vi "Query & Delete RTSeq Test Data.vi"(8 "Error In":errorcluster, 11 "RT Seq Ref In":refnum<k24>) -> (0 "Error Out":errorcluster, 1 "Parameters":refnum<k24>[](array[refnum]), 3 "RT Seq Ref Out":refnum<k24>, 5 "1 CSVs Tests":T1)   [LabVIEW 2011]
uses:
  NationalInstruments.VeriStand.RealTimeSequenceDefinitionApi
  Controls/CSVs Tests Data.ctl
  Controls/Test Column Data.ctl
  NationalInstruments.VeriStand.DataTypes
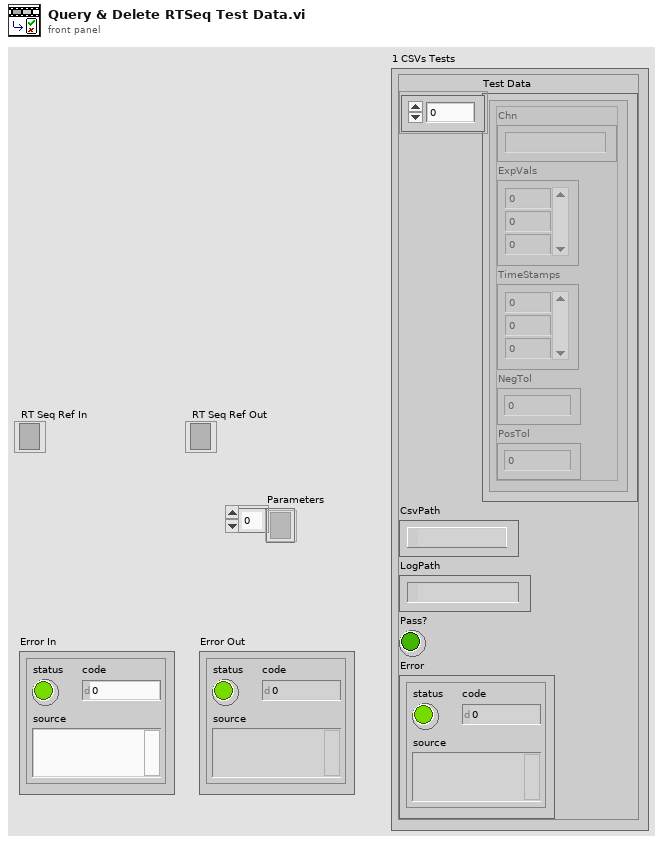
[diagram p1: front panel]
types:
  T1 = typedef "CSVs Tests Data.ctl" = cluster{"Test Data":T2[], "CsvPath":path, "LogPath":path, "Pass?":bool, "Error":errorcluster}
  T2 = typedef "Test Column Data.ctl" = cluster{"Chn":string, "ExpVals":dbl[], "TimeStamps":i64[], "NegTol":dbl, "PosTol":dbl}
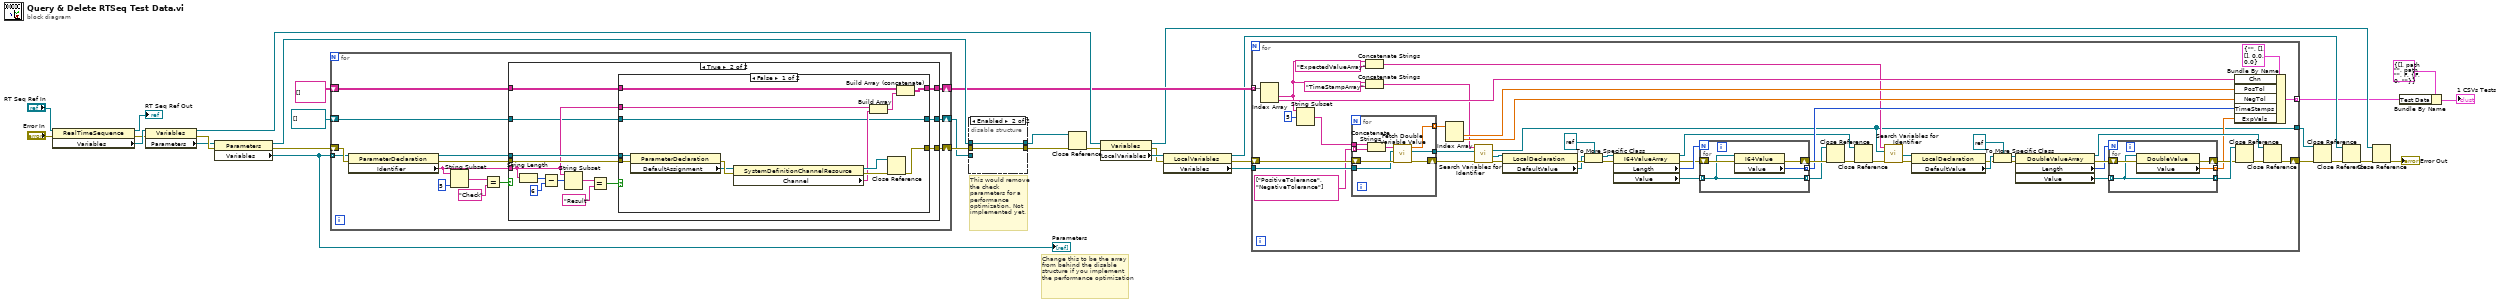
[diagram p0: block diagram]
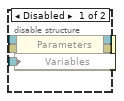
[diagram p2: hidden frame]
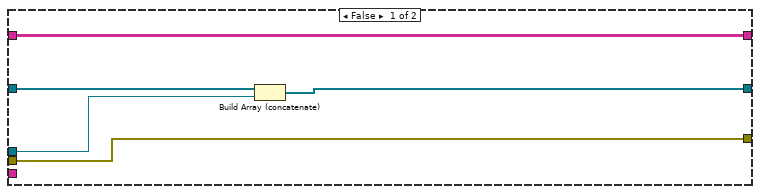
[diagram p3: hidden frame]
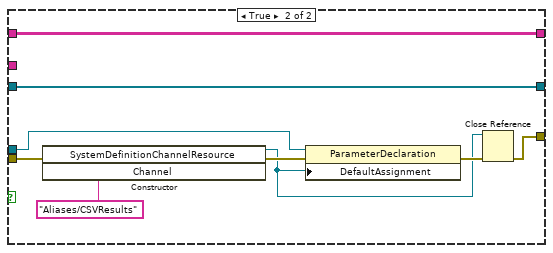
[diagram p4: hidden frame]
diagram:
  # "Change this to be the array from behind the disable structure if you implement the performance optimization"
  # "This would remove the check parameters for a performance optimization. Not implemented yet."
  n1 = property class="RealTimeSequence"(reference="RT Seq Ref In", error in="Error In") -> (reference out=→"RT Seq Ref Out":refnum<k24>, error out=w32:errorcluster, "Variables"=w33:refnum<k24>)
  n2 = property class="Variables"(reference=w33, error in=w32) -> (reference out=w17:refnum<k24>, error out=w28:errorcluster, "Parameters"=w25:refnum<k24>)
  n3 = property class="Parameters"(reference=w25, error in=w28) -> (reference out=w21:refnum<k24>, error out=w27:errorcluster, "Variables"=w20:refnum<k24>[])
  "Parameters" <- w20
  n4 = for {
    tunnel: w20 -> [w46] mode=indexing
    shift-right: [w34] -> w23
    shift-left: w27 -> [w47]
    shift-right: [w37] -> w16
    shift-left: string[][] [] -> [w38]
    shift-right: [w35] -> w22
    shift-left: refnum<k24>[] [] -> [w36]
    n5 = property class="ParameterDeclaration"(reference=w46, error in=w47) -> (reference out=w40:refnum<k24>, error out=w42:errorcluster, "Identifier"=w39:string)
    n6 = String Subset(string=w39, length (rest)=5 ("length (rest)")) -> (substring=w44:string)  [unwired: 1 in]
    n7 = Equal?(x=w44, y="Check") -> (x = y?=w41:bool)
    n8 = case shown="True" w41 {
      tunnel: w42 -> [w51 w60]
      tunnel: w40 -> [w49 w59]
      tunnel: w39 -> [_ w56]
      tunnel: w38 -> [w52 w58]
      tunnel: [w52 w57] -> w37
      tunnel: w36 -> [w50 w55]
      tunnel: [w48 w54] -> w35
      tunnel: [w51 w53] -> w34
      frame False {
        n9 = Build Array (concatenate)(w50, w49) -> (w48:refnum<k24>[])
      }
      frame True {
        n10 = String Length(string=w56) -> (length=w66:i32)
        n11 = Subtract(x=w66, y=6) -> (x-y=w64:i32)
        n12 = String Subset(string=w56, offset (0)=w64) -> (substring=w63:string)  [unwired: 1 in]
        n13 = Equal?(x=w63, y="Result") -> (x = y?=w61:bool)
        n14 = case shown="False" w61 {
          tunnel: w60 -> [w79 w86]
          tunnel: w59 -> [w78 w84]
          tunnel: w58 -> [w75 w88]
          tunnel: [w74 w88] -> w57
          tunnel: [w71 w80] -> w53
          tunnel: w56 -> [w69 _]
          tunnel: w55 -> [w67 w87]
          tunnel: [w67 w87] -> w54
          frame False {
            n15 = property class="ParameterDeclaration"(reference=w78, error in=w79) -> (error out=w77:errorcluster, "DefaultAssignment"=w76:refnum<k24>)  [unwired: 1 out]
            n16 = property class="SystemDefinitionChannelResource"(reference=w76, error in=w77) -> (reference out=w72:refnum<k24>, error out=w73:errorcluster, "Channel"=w68:string)
            n17 = Build Array(w69, w68) -> (w70:string[])
            n18 = Close Reference(reference=w72, error in (no error)=w73) -> (error out=w71:errorcluster)
            n19 = Build Array (concatenate)(w75, w70) -> (w74:string[][])
          }
          frame True {
            n20 = constructor class="SystemDefinitionChannelResource"(error in=w86, "Channel"="Aliases/CSVResults" ("y")) -> (reference out=w81:refnum<k24>, error out=w85:errorcluster)  [unwired: 2 in, 2 out]
            n21 = property class="ParameterDeclaration"(reference=w84, error in=w85, "DefaultAssignment"=w81) -> (error out=w82:errorcluster)  [unwired: 1 out]
            n22 = Close Reference(reference=w81, error in (no error)=w82) -> (error out=w80:errorcluster)
          }
        }
      }
    }
  }
  n23 = disable-structure shown="Enabled" {
    disable-tunnel: w23 -> [w93 w95]
    disable-tunnel: w22 -> [w92 _]
    disable-tunnel: w21 -> [w91 w94]
    disable-tunnel: [w90 w95] -> w4
    disable-tunnel: [w89 w94] -> w19
    frame Disabled {
      n24 = property class="Parameters"(reference=w91, error in=w93, "Variables"=w92) -> (reference out=w89:refnum<k24>, error out=w90:errorcluster)
    }
    frame Enabled {
    }
  }
  n25 = Close Reference(reference=w19, error in (no error)=w4) -> (error out=w18:errorcluster)
  n26 = property class="Variables"(reference=w17, error in=w18) -> (reference out=w6:refnum<k24>, error out=w14:errorcluster, "LocalVariables"=w15:refnum<k24>)
  n27 = property class="LocalVariables"(reference=w15, error in=w14) -> (reference out=w7:refnum<k24>, error out=w12:errorcluster, "Variables"=w13:refnum<k24>[])
  n28 = for {
    tunnel: w16 -> [w146] mode=indexing
    tunnel: w13 -> [w144]
    shift-right: [w97] -> w11
    shift-left: w12 -> [w147]
    tunnel: [w130] -> w2 mode=indexing
    tunnel: [w96] -> w10
    n29 = Index Array(array=w146) -> (element #1=w131:string, element #2=w142:string)  [unwired: 2 in]
    n30 = String Subset(string=w131, offset (0)=5) -> (substring=w141:string)  [unwired: 1 in]
    n31 = for {
      tunnel: w144 -> [w161]
      tunnel: w141 -> [w160]
      shift-right: [w158] -> w136
      shift-left: w147 -> [w163]
      tunnel: string[] ["PositiveTolerance", "NegativeTolerance"] -> [w159] mode=indexing
      tunnel: [w157] -> w135
      tunnel: [w156] -> w139 mode=indexing
      n32 = Concatenate Strings(w160, w159) -> (w162:string)
      n33 = call "Fetch Double Variable Value.vi"("error in (no error)"=w163, "Variables"=w161, "Identifier"=w162) -> ("error out"=w158:errorcluster, "Variables dup"=w157:refnum<k24>[], "Value"=w156:dbl)  [unwired: 6 in]
    }
    n34 = Concatenate Strings(w131, "ExpectedValueArray" ("string")) -> (w113:string)
    n35 = Concatenate Strings(w131, "TimeStampArray" ("string")) -> (w133:string)
    n36 = Index Array(array=w139) -> (element #1=w138:dbl, element #2=w137:dbl)  [unwired: 2 in]
    n37 = call "Search Variables for Identifier.vi"("error in (no error)"=w136, "Variables"=w135, "Identifier"=w133) -> ("error out"=w124:errorcluster, "Found Variable"=w123:refnum<k24>, "Variables dup"=w96:refnum<k24>[])  [unwired: 6 in]
    n38 = property class="LocalDeclaration"(reference=w123, error in=w124) -> (error out=w129:errorcluster, "DefaultValue"=w128:refnum<k24>)  [unwired: 1 out]
    n39 = To More Specific Class(target class=refnum<k24> refnum, reference=w128, error in=w129) -> (specific class reference=w125:refnum<k24>, error out=w126:errorcluster)
    n40 = property class="I64ValueArray"(reference=w125, error in=w126) -> (reference out=w115:refnum<k24>, error out=w120:errorcluster, "Length"=w121:i64, "Value"=w122:refnum<k24>[])
    n41 = for {
      N: w121 -> [_]
      tunnel: w122 -> [w152] mode=indexing
      shift-right: [w154] -> w119
      shift-left: w120 -> [w155]
      tunnel: [w153] -> w118 mode=indexing
      tunnel: [w152] -> w117 mode=indexing
      n42 = property class="I64Value"(reference=w152, error in=w155) -> (error out=w154:errorcluster, "Value"=w153:i64)  [unwired: 1 out]
    }
    n43 = Close Reference(reference=w117, error in (no error)=w119) -> (error out=w116:errorcluster)
    n44 = Close Reference(reference=w115, error in (no error)=w116) -> (error out=w114:errorcluster)
    n45 = call "Search Variables for Identifier.vi"("error in (no error)"=w114, "Variables"=w96, "Identifier"=w113) -> ("error out"=w99:errorcluster, "Found Variable"=w100:refnum<k24>)  [unwired: 6 in, 1 out]
    n46 = property class="LocalDeclaration"(reference=w100, error in=w99) -> (error out=w101:errorcluster, "DefaultValue"=w102:refnum<k24>)  [unwired: 1 out]
    n47 = To More Specific Class(target class=refnum<k24> refnum, reference=w102, error in=w101) -> (specific class reference=w105:refnum<k24>, error out=w104:errorcluster)
    n48 = property class="DoubleValueArray"(reference=w105, error in=w104) -> (reference out=w112:refnum<k24>, error out=w108:errorcluster, "Length"=w107:i64, "Value"=w106:refnum<k24>[])
    n49 = for {
      N: w107 -> [_]
      tunnel: w106 -> [w148] mode=indexing
      shift-right: [w150] -> w109
      shift-left: w108 -> [w151]
      tunnel: [w149] -> w98 mode=indexing
      tunnel: [w148] -> w110 mode=indexing
      n50 = property class="DoubleValue"(reference=w148, error in=w151) -> (error out=w150:errorcluster, "Value"=w149:dbl)  [unwired: 1 out]
    }
    n51 = Bundle By Name(cluster=T2 {"Chn"="", "ExpVals"=[], "TimeStamps"=[], "NegTol"=0.0, "PosTol"=0.0} ("ValueTest"), "Chn"=w142, "PosTol"=w138, "NegTol"=w137, "TimeStamps"=w118, "ExpVals"=w98) -> (w130:T2)
    n52 = Close Reference(reference=w110, error in (no error)=w109) -> (error out=w111:errorcluster)
    n53 = Close Reference(reference=w112, error in (no error)=w111) -> (error out=w97:errorcluster)
  }
  n54 = Close Reference(reference=w10, error in (no error)=w11) -> (error out=w9:errorcluster)
  n55 = Close Reference(reference=w7, error in (no error)=w9) -> (error out=w8:errorcluster)
  n56 = Close Reference(reference=w6, error in (no error)=w8) -> (error out=→"Error Out":errorcluster)
  n57 = Bundle By Name(cluster=T1 {"Test Data"=[], "CsvPath"=path "", "LogPath"=path "", "Pass?"=FALSE, "Error"={"status"=FALSE, "code"=0, "source"=""}} ("1 CSVs Tests"), "Test Data"=w2) -> (→"1 CSVs Tests":T1)
